vi "ND2_GetFirstFrame.vi"(8 "error in (no error)":errorcluster, 11 "FilePath":path=path "C:/Users/VirtualUser/Desktop/EPA Image Processing/test images/150806-005.nd2") -> (0 "error out":errorcluster, 1 "LIMLOCALMETADATA":T1 {"dTimeMSec" format="%.2f"}, 3 "Image out":T2)   [LabVIEW 2014, in "ND2_Reader_32.lvlib"]
uses:
  ND2_Reader_32.lvlib
  <vilib>/vision/Image Controls.llb/IMAQ Image.ctl
  controls/cluster_LIMLOCALMETADATA.ctl
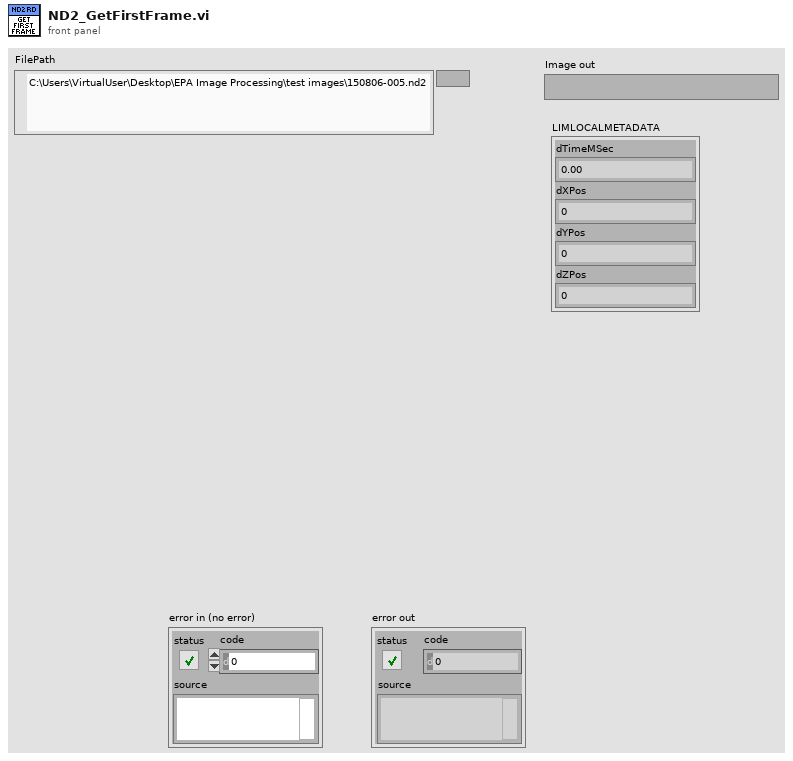
[diagram p1: front panel]
types:
  T1 = typedef "cluster_LIMLOCALMETADATA.ctl" = cluster{"dTimeMSec":dbl, "dXPos":dbl, "dYPos":dbl, "dZPos":dbl}
  T2 = typedef "IMAQ Image.ctl" = refnum<image>
  T3 = typedef "Image Type" = u32
  T4 = typedef "cluster_LIMPICTURE.ctl" = cluster{"uiWidth":u32, "uiHeight":u32, "uiBitsPerComp":u32, "uiComponents":u32, "uiWidthBytes":u32, "uiSize":u32, "pImageData":u32}
  T5 = typedef "numeric_LIMFILEHANDLE.ctl" = i32
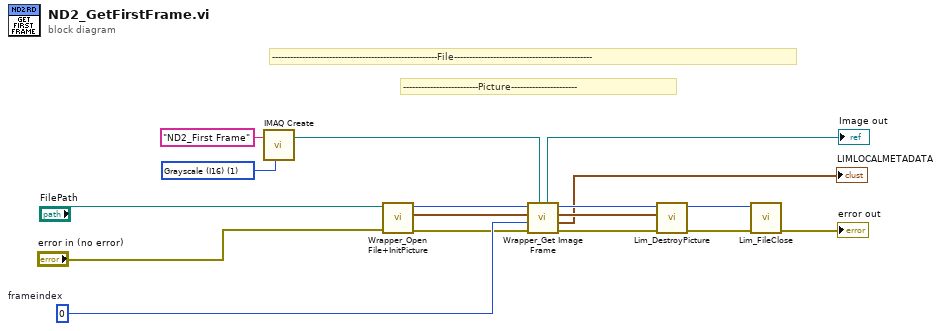
[diagram p0: block diagram]
diagram:
  w11 = 0  # frameindex
  w13 = T3 1 items=["Grayscale (U8)", "Grayscale (I16)", "Grayscale (SGL)", "Complex (CSG)", "RGB (U32)", "HSL (U32)", "RGB (U64)", "Grayscale (U16)"] ("Image Type")
  # "-------------------------Picture----------------------"
  # "-------------------------------------------------------File----------------------------------------------"
  n1 = call "IMAQ Create"("Image Name"="ND2_First Frame", "Image Type"=w13) -> ("New Image"=w10:T2)  [unwired: 3 in, 1 out]
  n2 = call "Wrapper_Open File+InitPicture.vi"("error in (no error)"="error in (no error)", "FilePath"="FilePath") -> ("error out"=w5:errorcluster, "LIMPICTUREout"=w1:T4, "hFile out"=w4:T5)  [unwired: 6 in, 1 out]
  n3 = call "Wrapper_Get Image Frame.vi"("Image Ref in"=w10, "error in (no error)"=w5, "frameindex in"=w11, "LIMPICTURE in"=w1, "hFile in"=w4) -> ("error out"=w15:errorcluster, "LIMLOCALMETADATA"=→"LIMLOCALMETADATA":T1, "LIMPICTURE out"=w7:T4, "hFile out"=w8:T5, "Image Ref out"=→"Image out":T2)  [unwired: 2 in]
  n4 = call "Lim_DestroyPicture.vi"("error in (no error)"=w15, "LIMPICTURE"=w7, "hFile in"=w8) -> ("error out"=w16:errorcluster, "hFile out"=w17:T5)  [unwired: 7 in]
  n5 = call "Lim_FileClose.vi"("error in (no error)"=w16, "hFile in"=w17) -> ("error out"=→"error out":errorcluster)  [unwired: 8 in, 1 out]
